vi "ResonanceAnalyzer.vi"() -> ()   [LabVIEW 2014]
uses:
  <vilib>/imath/engines/lvmath2/RunTimeEngine/Managers/WorkSpace/UID Generator.vi
  <vilib>/imath/engines/lvmath2/RunTimeEngine/RangeToken/NIMS_Range.vi
  <instcachedir>/0/NIMS_Range_9BCE657718DF4976A877346C61F22738.lvgen/NIMS_Range_9BCE657718DF4976A877346C61F22738_000.vi
  <vilib>/imath/engines/lvmath2/RunTimeEngine/RunTimeType/NIMS_RunTimeType_From StrictType (excl LVString).vi
  <instcachedir>/0/NIMS_RunTimeType_From StrictType (excl LVString)_15A5391EEA9C4AACB9955AC755B83D29.lvgen/NIMS_RunTimeType_From StrictType (excl LVString)_15A5391EEA9C4AACB9955AC755B83D29_000.vi
  <vilib>/imathl/engines/lvmath/Functions/Error Handling/Create Error.vi
  <vilib>/imath/engines/lvmath2/RunTimeEngine/LocalVariableDefStatement/MC_LocalVariableDefStatement_Display.vi
  <vilib>/imath/engines/lvmath2/RunTimeEngine/ArithmeticOperatorToken/NIMS_ArithmeticOperator_minus.vi
  <instcachedir>/0/NIMS_ArithmeticOperator_minus_39C0593E74DA4138ACA2AB742906488D.lvgen/NIMS_ArithmeticOperator_minus_39C0593E74DA4138ACA2AB742906488D_003.vi
  <vilib>/imath/engines/lvmath2/RunTimeEngine/BuiltInFunctions/length/NIMS_length(GV).vi
  <instcachedir>/0/NIMS_length(GV)_08A3D13377FD4E4B96F5795FBF3698FA.lvgen/NIMS_length(GV)_08A3D13377FD4E4B96F5795FBF3698FA_001.vi
  <vilib>/imath/engines/lvmath2/RunTimeEngine/BuiltInFunctions/randnormal/NIMS_randnormal(1,I32).vi
  <vilib>/imath/engines/lvmath2/RunTimeEngine/ErrorHandling/NIMS_Error From Error Code.vi
  <vilib>/imath/engines/lvmath2/RunTimeEngine/ArithmeticOperatorToken/NIMS_ArithmeticOperator_plus.vi
  <instcachedir>/0/NIMS_ArithmeticOperator_plus_48D6EAACA5D645B09F7EC9C016C2DEA8.lvgen/NIMS_ArithmeticOperator_plus_48D6EAACA5D645B09F7EC9C016C2DEA8_000.vi
  <vilib>/imath/engines/lvmath2/RunTimeEngine/Managers/SymbolTable/Clear UID.vi
  <vilib>/imath/engines/lvmath2/RunTimeEngine/NodeEndStatement/NIMS_NodeEndStatement_Output.vi
  <instcachedir>/0/NIMS_NodeEndStatement_Output_53EC0D466D134D7ABD903AC30B43404B.lvgen/NIMS_NodeEndStatement_Output_53EC0D466D134D7ABD903AC30B43404B_000.vi
  <instcachedir>/0/NIMS_NodeEndStatement_Output_53EC0D466D134D7ABD903AC30B43404B.lvgen/NIMS_NodeEndStatement_Output_53EC0D466D134D7ABD903AC30B43404B_005.vi
  <vilib>/imath/engines/lvmath2/RunTimeEngine/ErrorHandling/NIMS_Finalize Error.vi
  <vilib>/imath/engines/lvmath2/RunTimeEngine/Managers/SymbolTable/NIMS_WorkSpace.lvlib
panel:
  out "XY Graph":cluster{"f":dbl[], "noisey_data":dbl[]}(graph)={"f"=[0.0, 2900.0, 2901.0, 2902.0, 2903.0, 2904.0, 2905.0, 2906.0, 2907.0, 2908.0, 2909.0, 2910.0, 2911.0, 2912.0, 2913.0, 2914.0, 2915.0, 2916.0, 2917.0, 2918.0, 2919.0, 2920.0, 2921.0, 2922.0, 2923.0, 2924.0, 2925.0, 2926.0, 2927.0, 2928.0, 2929.0, 2930.0, 2931.0, 2932.0, 2933.0, 2934.0, 2935.0, 2936.0, 2937.0, 2938.0, 2939.0, 2940.0, 2941.0, 2942.0, 2943.0, 2944.0, 2945.0, 2946.0, 2947.0, 2948.0, 2949.0, 2950.0, 2951.0, 2952.0, 2953.0, 2954.0, 2955.0, 2956.0, 2957.0, 2958.0, 2959.0, 2960.0, 2961.0, 2962.0, 2963.0, 2964.0, 2965.0, 2966.0, 2967.0, 2968.0, 2969.0, 2970.0, 2971.0, 2972.0, 2973.0, 2974.0, 2975.0, 2976.0, 2977.0, 2978.0, 2979.0, 2980.0, 2981.0, 2982.0, 2983.0, 2984.0, 2985.0, 2986.0, 2988.0, 2989.0, 2990.0, 2991.0, 2992.0, 2993.0, 2994.0, 2995.0, 2996.0, 2997.0, 2998.0, 2999.0, 3000.0, 3001.0, 3002.0, 3003.0, 3004.0, 3005.0, 3006.0, 3007.0, 3008.0, 3009.0, 3010.0, 3011.0, 3012.0, 3013.0, 3014.0, 3015.0, 3016.0, 3017.0, 3018.0, 3019.0, 3020.0, 3021.0, 3022.0, 3023.0, 3024.0, 3025.0, 3026.0, 3027.0, 3028.0, 3029.0, 3030.0, 3031.0, 3032.0, 3033.0, 3034.0, 3035.0, 3036.0, 3037.0, 3038.0, 3039.0, 3040.0, 3041.0, 3042.0, 3043.0, 3044.0, 3045.0, 3046.0, 3047.0, 3048.0, 3049.0, 3050.0, 3051.0, 3052.0, 3053.0, 3054.0, 3055.0, 3056.0, 3057.0, 3058.0, 3059.0, 3060.0, 3061.0, 3062.0, 3063.0, 3064.0, 3065.0, 3066.0, 3067.0, 3068.0, 3069.0, 3070.0, 3071.0, 3072.0, 3073.0, 3074.0, 3075.0], "noisey_data"=[0.0, -37.70338, -37.61902, -37.77387, -37.79925, -37.82478, -37.83581, -37.84899, -37.85769, -37.87101, -37.8669, -37.87504, -37.87234, -37.86832, -37.86504, -37.8603, -37.84629, -37.82555, -37.7994, -37.78175, -37.75951, -37.73503, -37.70237, -37.66082, -37.62423, -37.5854, -37.53785, -37.50966, -37.46281, -37.40161, -37.34955, -37.28907, -37.23375, -37.16185, -37.08815, -37.00953, -36.93567, -36.85559, -36.76932, -36.66591, -36.57793, -36.47671, -36.3756, -36.26493, -36.15583, -36.03271, -35.9025, -35.77349, -35.64244, -35.49688, -35.34783, -35.19521, -35.03437, -34.86675, -34.69336, -34.50751, -34.39355, -34.19773, -34.01007, -33.80534, -33.59208, -33.37763, -33.15881, -32.91547, -32.66409, -32.40725, -32.13479, -31.86032, -31.56244, -31.25799, -30.93439, -30.59497, -30.24431, -29.87801, -29.48651, -29.07503, -28.64193, -28.18302, -27.69297, -27.16537, -26.6112, -26.02447, -25.3938, -24.72038, -24.00837, -23.52048, -22.76489, -21.98091, -21.1649, -19.56535, -18.87876, -18.37747, -18.13793, -18.20447, -18.56283, -19.15075, -19.88533, -20.69376, -21.52182, -22.33604, -23.12045, -23.86634, -24.57676, -25.24494, -25.87668, -26.47212, -27.03527, -27.57211, -28.07746, -28.55822, -29.01191, -29.45127, -29.86245, -30.26642, -30.50621, -30.85414, -31.19036, -31.50529, -31.81557, -32.1023, -32.38428, -32.65338, -32.91483, -33.16338, -33.3931, -33.62432, -33.84874, -34.06179, -34.26566, -34.46412, -34.65738, -34.84016, -35.02199, -35.18415, -35.35683, -35.51453, -35.66286, -35.82195, -35.96707, -36.09568, -36.22869, -36.36305, -36.48085, -36.55571, -36.67646, -36.78197, -36.88595, -36.99335, -37.07483, -37.16822, -37.26067, -37.33494, -37.41554, -37.49919, -37.57867, -37.63455, -37.69278, -37.75796, -37.82405, -37.87578, -37.92458, -37.96844, -38.01212, -38.0604, -38.09456, -38.1447, -38.17476, -38.19251, -38.22557, -38.25037, -38.26333, -38.2586, -38.29777, -38.2975, -38.30544, -38.31027]}
  in  "Tab Control":enum32{"Simulation", "Experiment"}(tab)=enum."Experiment"
  in  "input cluster":T1
  in  "file path (use dialog)":path=path "C:/Users/davidb52/Desktop/week6/output.txt"
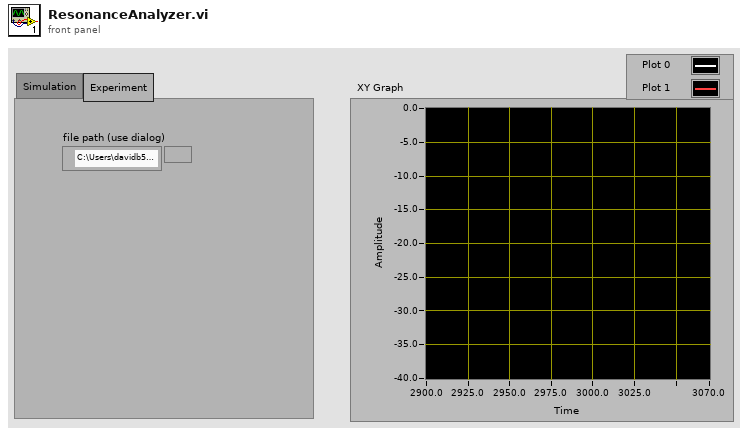
[diagram p1: front panel]
types:
  T1 = cluster{"Q":dbl, "Center Frequency":dbl, "Start Frequency":dbl, "End Frequency":dbl, "df":dbl, "Noise Level":dbl}
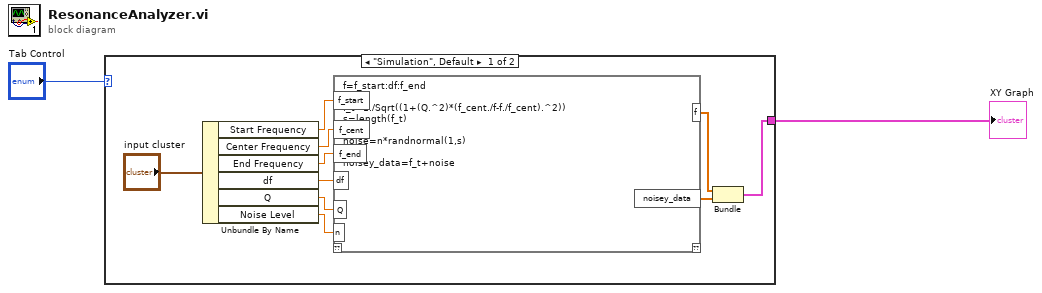
[diagram p0: block diagram]
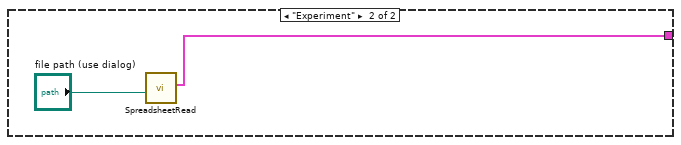
[diagram p2: hidden frame]
diagram:
  n1 = case shown="\"Simulation\", Default" "Tab Control" {
    tunnel: [w3 w177] -> w1
    frame "Simulation", Default {
      n2 = Unbundle By Name("input cluster") -> ("Start Frequency"=w12:dbl, "Center Frequency"=w11:dbl, "End Frequency"=w10:dbl, "df"=w9:dbl, "Q"=w8:dbl, "Noise Level"=w7:dbl)
      n3 = mathscript code="f=f_start:df:f_end\n\nf_t=1./Sqrt((1+(Q.^2)*(f_cent./f-f./f_cent).^2))\ns=length(f_t)\n\nnoise=n*randnormal(1,s)\n\nnoisey_data=f_t+noise"("Q"=w8, "f_cent"=w11, "f_start"=w12, "f_end"=w10, "df"=w9, "n"=w7) -> ("f"=w5:dbl[], "noisey_data"=w4:cdb[])  [unwired: 1 in, 1 out]
      n4 = Bundle("f"=w5, "noisey_data"=w4) -> (w3:cluster{"f":dbl[], "noisey_data":cdb[]})  [unwired: 1 in]
    }
    frame "Experiment" {
      n5 = call "SpreadsheetRead.vi"("file path (use dialog)"="file path (use dialog)") -> ("output cluster"=w177:cluster{dbl[], dbl[]})  [unwired: 10 in]
    }
  }
  "XY Graph" <- w1
